vi "test.vi"() -> ()   [LabVIEW 2014]
uses:
  Controls/4 Track Audio.ctl
  Controls/Audio In.ctl
  <vilib>/myRIO/Instrument Drivers/Onboard IO/AudioOut Block/typedefs/AudioOut Block Reference.ctl
  <vilib>/myRIO/Common/Instrument Driver Framework/Utilities/typedefs/myRIO Generic Hardware Reference.ctl
  <vilib>/myRIO/Common/Instrument Driver Framework/Utilities/typedefs/Hardware Version Enum.ctl
  <vilib>/myRIO/Common/Instrument Driver Framework/Utilities/typedefs/myRIO v1.0 Reference.ctl
  <vilib>/myRIO/Common/Instrument Driver Framework/Utilities/typedefs/Generic FPGA Reference.ctl
  <vilib>/myRIO/Common/Instrument Driver Framework/myRIO v1.0/AudioOut Block/typedefs/AudioOut Block Channels List.ctl
  <vilib>/myRIO/Common/Instrument Driver Framework/myRIO v1.0/AudioOut Block/typedefs/AudioOut Block Channels Enum.ctl
  <vilib>/myRIO/Common/Instrument Driver Framework/Utilities/typedefs/Analog Scaling Constants.ctl
  <vilib>/userdefined/High Color/nirio_resource_hc.ctl
  <vilib>/myRIO/Common/Instrument Driver Framework/Utilities/vis/Is FPGA Ref Available.vi
  <vilib>/myRIO/Common/Instrument Driver Framework/myRIO v1.0/AudioOut Block/vis/myRIO v1.1 Open Throughput AudioOut (N Samples).vi
  <vilib>/myRIO/Instrument Drivers/Onboard IO/AudioOut Block/vis/Write.vi
  <vilib>/myRIO/Common/Instrument Driver Framework/Utilities/vis/Validate Channels.vi
  <vilib>/Utility/VariantDataType/GetNumericInfo.vi
  <vilib>/Utility/error.llb/Error Cluster From Error Code.vi
  <vilib>/myRIO/Common/Instrument Driver Framework/myRIO v1.0/myRIO v1.1 Open Throughput.vi
  <vilib>/myRIO/Common/Instrument Driver Framework/myRIO v1.0/AudioOut Block/vis/myRIO v1.0 Get Scaling Constants AudioOut Block.vi
  <vilib>/myRIO/Common/Instrument Driver Framework/myRIO v1.0/AudioOut Block/vis/myRIO v1.0 Reserve AudioOut Block.vi
  <vilib>/myRIO/Common/Instrument Driver Framework/myRIO v1.0/Resource Manager/vis/myRIO v1.0 Open Writing DMA.vi
  <vilib>/myRIO/Common/Instrument Driver Framework/myRIO v1.0/myRIO v1.0 Close.vi
  <vilib>/myRIO/Common/Instrument Driver Framework/myRIO v1.0/AudioOut Block/vis/myRIO v1.0 AudioOut Block Write.vi
  <vilib>/myRIO/Express VI/Onboard IO/AudioOut/AudioOut Express VI.xnode
  <vilib>/myRIO/Instrument Drivers/Onboard IO/AudioOut Block/vis/myRIO AudioOut N Samples Open.xnode
  <vilib>/myRIO/Instrument Drivers/Onboard IO/AudioOut Block/AudioOut Block.lvlib
panel:
  out "error out":errorcluster
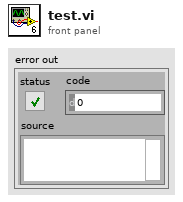
[diagram p1: front panel]
types:
  T1 = typedef "4 Track Audio.ctl" = cluster{"Track 0":T2, "Track 1":T2, "Track 2":T2, "Track 3":T2}
  T2 = typedef "Audio In.ctl" = cluster{"AudioIn/Left (N Samples)":dbl[], "AudioIn/Right (N Samples)":dbl[]}
  T3 = typedef "AudioOut Block.lvlib/AudioOut Block Reference.ctl" = cluster{"myRIO Reference":T4, "AudioOut (N Samples) Channels List":T8, "AudioOut (N Samples) Scaling Constants List":T10[]}
  T4 = typedef "myRIO Generic Hardware Reference.ctl" = cluster{"myRIO Model":T5, "myRIO Hardware Reference":T6}
  T5 = typedef "Hardware Version Enum.ctl" = enum16{"Unknown", "myRIO-1900", "myRIO-1950"}
  T6 = typedef "myRIO v1.0 Reference.ctl" = cluster{"Generic FPGA Reference":T7, "Allow multiple opens":bool}
  T7 = typedef "Generic FPGA Reference.ctl" = refnum<k20>
  T8 = typedef "AudioOut Block Channels List.ctl" = T9[]
  T9 = typedef "AudioOut Block Channels Enum.ctl" = enum16{"Not Connected", "AudioOut/Left (N Samples)", "AudioOut/Right (N Samples)"}
  T10 = typedef "Analog Scaling Constants.ctl" = cluster{"LSB Weight (Volts)":dbl, "Offset (Volts)":dbl, "Signed?":bool}
  T11 = typedef "nirio_resource_hc.ctl" = tag
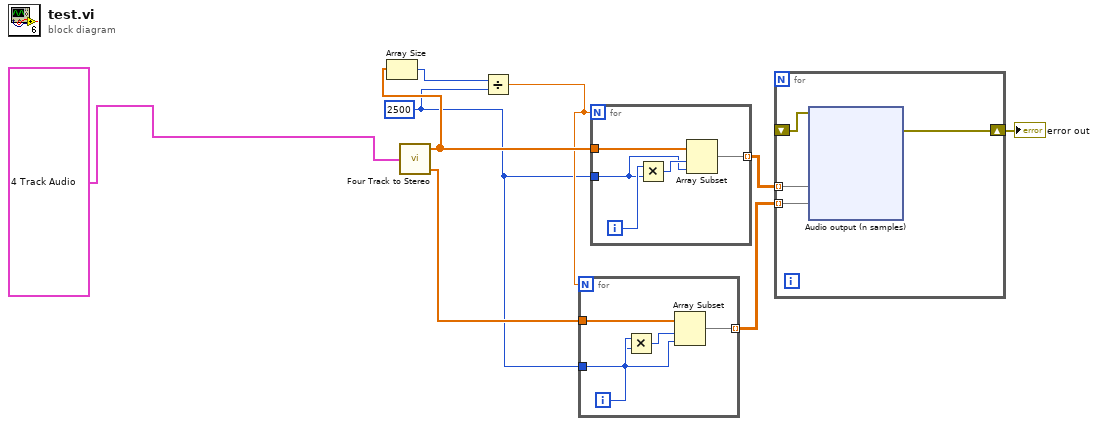
[diagram p0: block diagram]
diagram:
  w3 = 2500
  n1 = call "Four Track to Stereo.vi"("4-Track Audio In"=T1 {"Track 0"={"AudioIn/Left (N Samples)"=array[205000 elements], "AudioIn/Right (N Samples)"=array[205000 elements]}, "Track 1"={"AudioIn/Left (N Samples)"=array[205000 elements], "AudioIn/Right (N Samples)"=array[205000 elements]}, "Track 2"={"AudioIn/Left (N Samples)"=array[205000 elements], "AudioIn/Right (N Samples)"=array[205000 elements]}, "Track 3"={"AudioIn/Left (N Samples)"=array[205000 elements], "AudioIn/Right (N Samples)"=array[205000 elements]}} ("4-Track Audio out")) -> ("Right Out"=w8:dbl[], "Left Out"=w5:dbl[])  [unwired: 3 in]
  n2 = Array Size(array=w5) -> (size(s)=w6:i32)
  n3 = Divide(x=w6, y=w3) -> (x/y=w4:dbl)
  n4 = for {
    N: w4 -> [_]
    tunnel: w8 -> [w14]
    tunnel: [w11] -> w7 mode=indexing
    tunnel: w3 -> [w10]
    i -> [w12]
    n5 = Multiply(x=w12, y=w10) -> (x*y=w13:i32)
    n6 = Array Subset(array=w14, index=w13, length=w10) -> (w11:dbl[])
  }
  n7 = for {
    N: w4 -> [_]
    tunnel: w5 -> [w19]
    tunnel: [w16] -> w9 mode=indexing
    tunnel: w3 -> [w15]
    i -> [w17]
    n8 = Multiply(x=w17, y=w15) -> (x*y=w18:i32)
    n9 = Array Subset(array=w19, index=w18, length=w15) -> (w16:dbl[])
  }
  n10 = for {
    tunnel: w9 -> [w23] mode=indexing
    tunnel: w7 -> [w22] mode=indexing
    shift-right: [w21] -> w2
    shift-left: _ -> [w20]
    n11 = xnode "Audio output (n samples)"("AudioOut/Left (N Samples)"=w23, "AudioOut/Right (N Samples)"=w22, "error in (no error)"=w20) -> ("error out"=w21:errorcluster)
  }
  "error out" <- w2
